vi "Run Test - Remove NaN Value (SubVI).vi"(11 "Array":dbl[](array[numeric])) -> (3 "Array out":dbl[](array[numeric]))   [LabVIEW 2019]
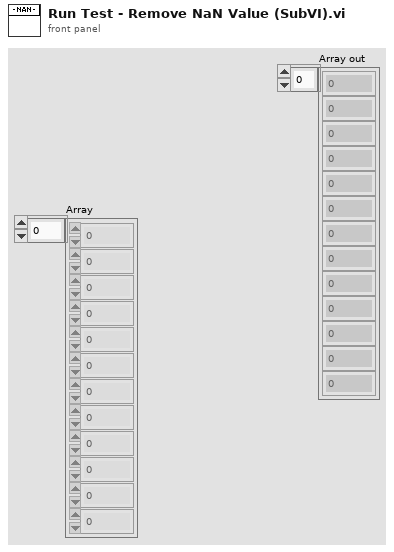
[diagram p1: front panel]
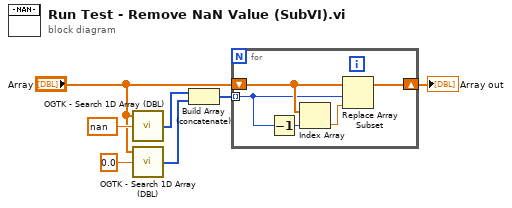
[diagram p0: block diagram]
diagram:
  n1 = call "OGTK - Search 1D Array (DBL).vi"("Array"="Array", "Element Data"=nan ("element")) -> ("Indices of Elements"=w4:i32[])  [unwired: 7 in]
  n2 = call "OGTK - Search 1D Array (DBL).vi"("Array"="Array", "Element Data"=0.0 ("element")) -> ("Indices of Elements"=w1:i32[])  [unwired: 7 in]
  n3 = Build Array (concatenate)(w4, w1) -> (w7:i32[])
  n4 = for {
    tunnel: w7 -> [w10] mode=indexing
    shift-right: [w8] -> w6
    shift-left: "Array" -> [w12]
    n5 = Decrement(x=w10) -> (x-1=w11:i32)
    n6 = Index Array(array=w12, index=w11) -> (element=w9:dbl)
    n7 = Replace Array Subset(array=w12, new element=w9, index=w10) -> (w8:dbl[])
  }
  "Array out" <- w6
